vi "Live Modification Dialog.vi"(11 "Front Panel Objects":refnum<vi>[](array[refnum])) -> ()   [LabVIEW 2019, in "LSS.lvlib"]
doc: "This dialog box can be used to help generate style sheets and observe their effect on the user interface. The editor will populate with the default values for each LSS style when an item from \"Available Properties\" is double clicked. \n\n<b>Inputs:</b>\n<b>Front Panel Objects</b> - Although the editor is setup to allow a user to select an active VI to edit, this input can be used to pass in Front Panel Objects if the references are already open when usinng this VI as a pop up dialog."
uses:
  LSS.lvlib
  Controls/Mode.ctl
panel:
  out "Error Out":errorcluster
  in  "Error In":errorcluster
  in  "Color Map":string
  in  "Editable VIs":i32[](listbox)
  in  "HEX":string
  in  "B":u32 max=255
  in  "G":u32 max=255
  in  "R":u32 max=255
  in  "Color Picker":u32(colorbox)
  in  "Clear":bool
  out "Applicable Controls":i32(listbox)
  in  "Available Properties":i32(listbox) caption="Available Properties\n(double click to add)"
  out "More Specific Identifiers":i32(listbox)
  out "More Generic Identifiers":i32(listbox)
  in  "Unique Identifiers":i32(listbox)
  in  "Load":bool
  in  "Save":bool
  in  "Apply":bool
  in  "LSS Editor":string
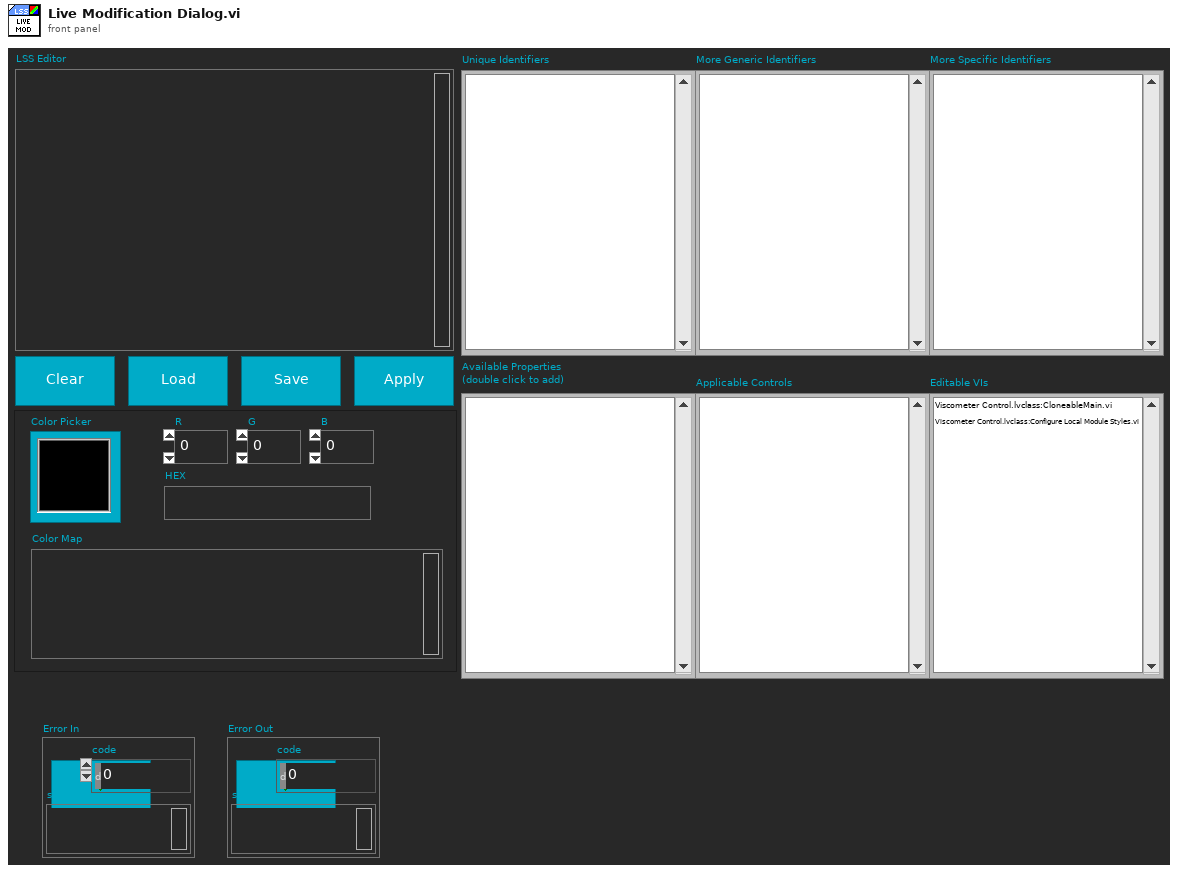
[diagram p1: front panel]
types:
  T1 = typedef "LSS.lvlib/Mode.ctl" = enum16{"Write", "Add", "Read"}
  T2 = typedef "LVPoint32TypeDef.ctl" = cluster{"Horizontal":i32, "Vertical":i32}
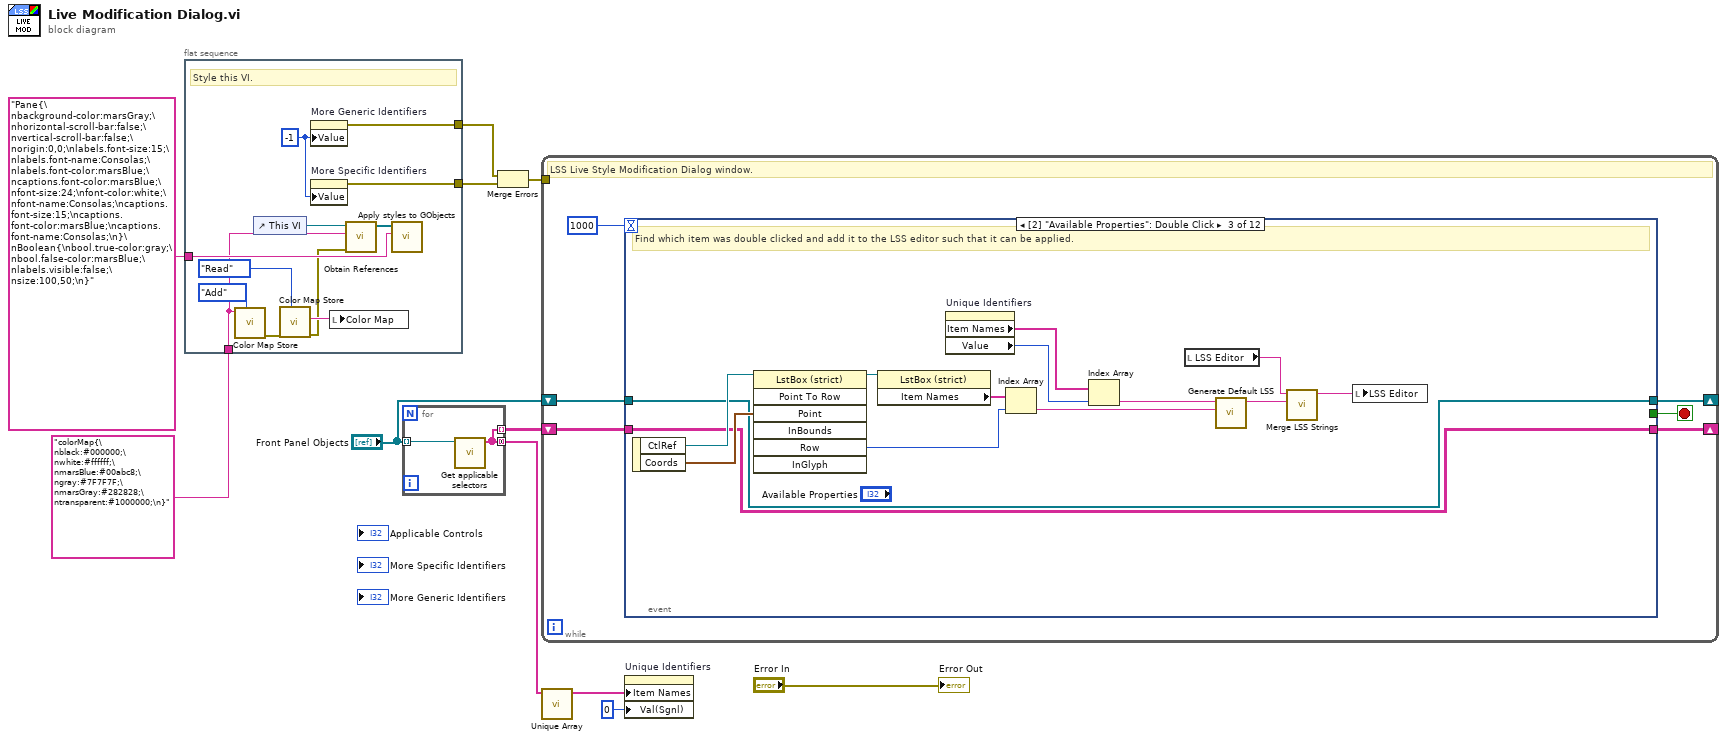
[diagram p0: block diagram]
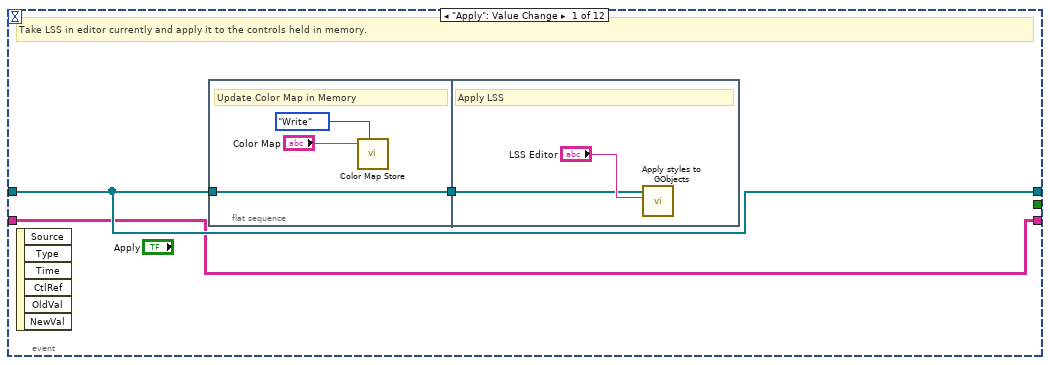
[diagram p2: hidden frame]
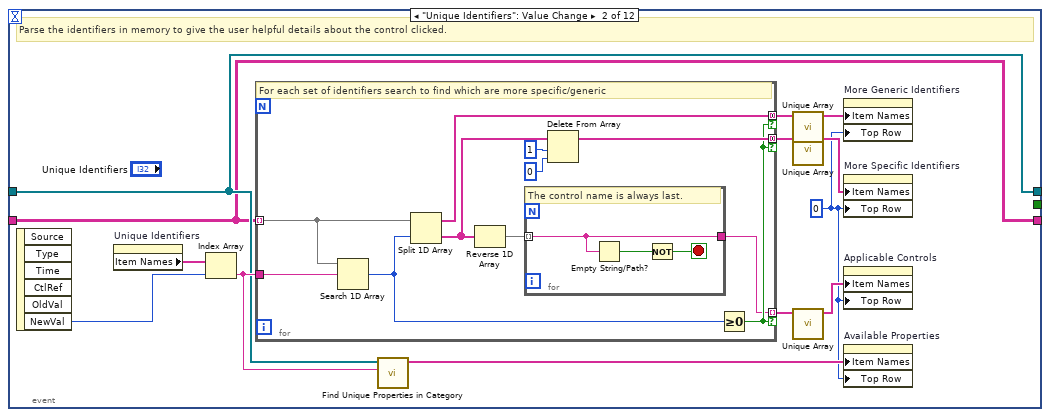
[diagram p3: hidden frame]
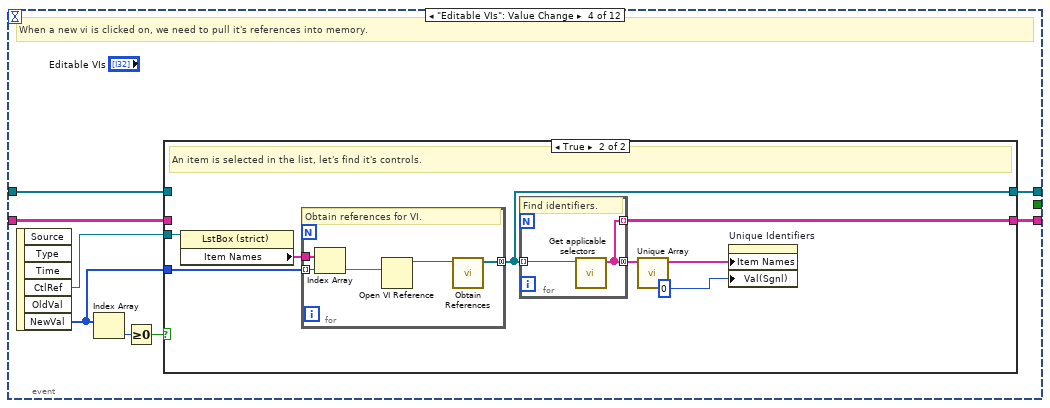
[diagram p4: hidden frame]
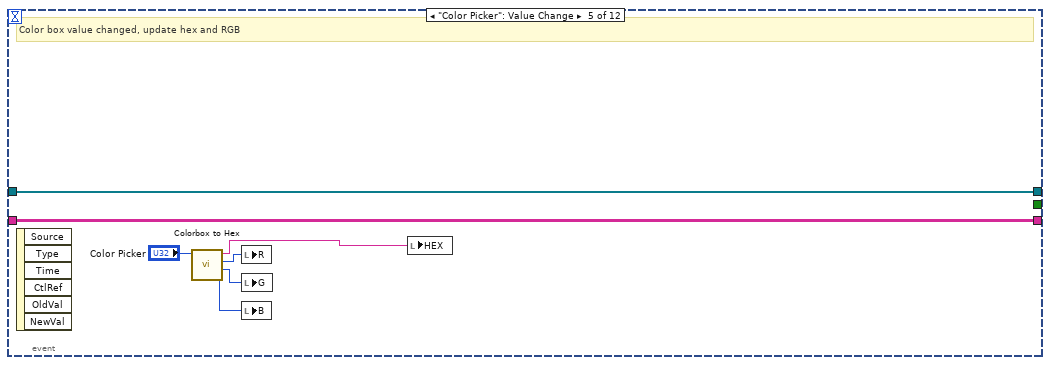
[diagram p6: hidden frame]
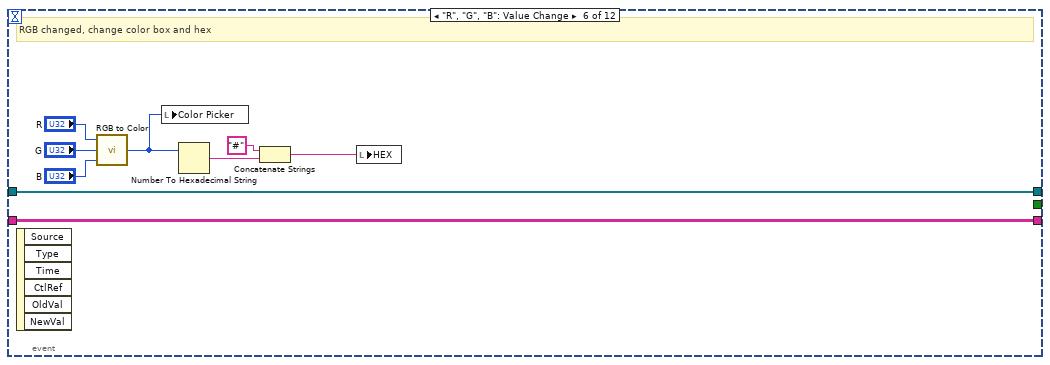
[diagram p7: hidden frame]
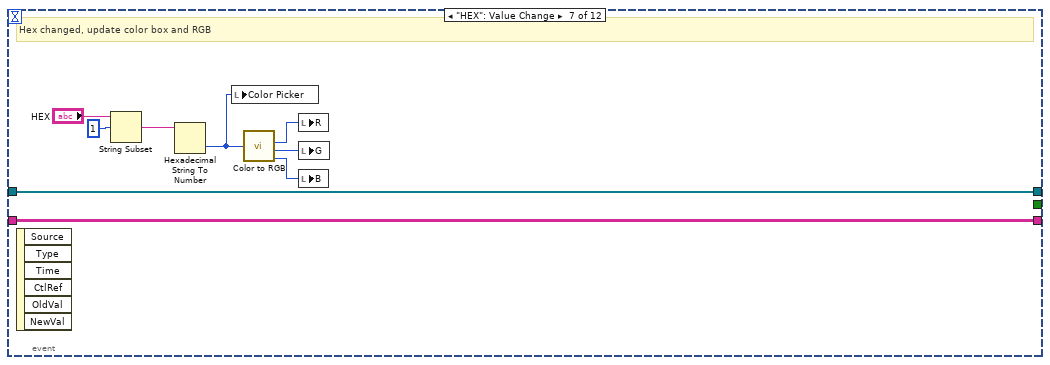
[diagram p8: hidden frame]
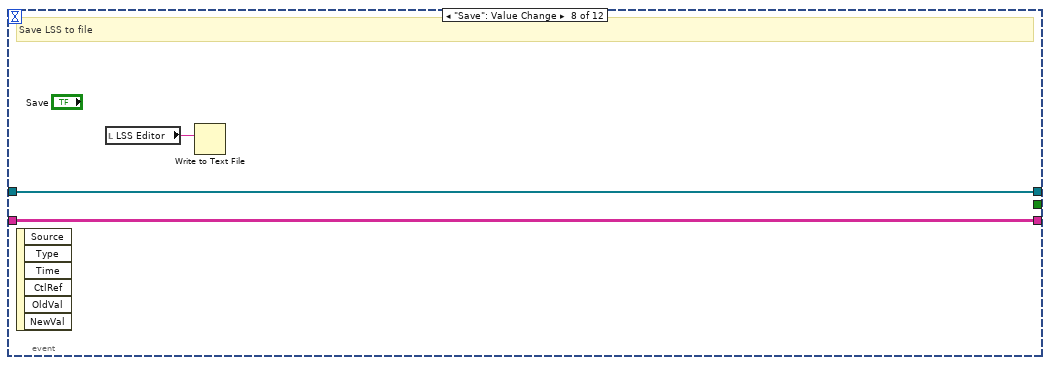
[diagram p9: hidden frame]
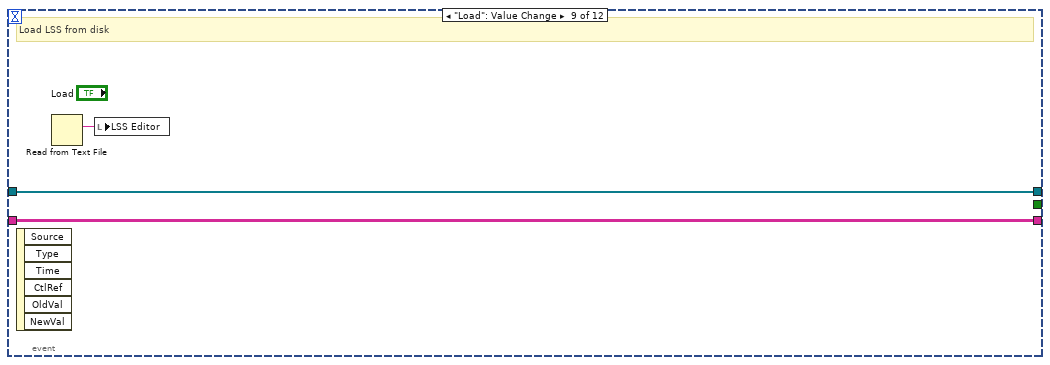
[diagram p10: hidden frame]
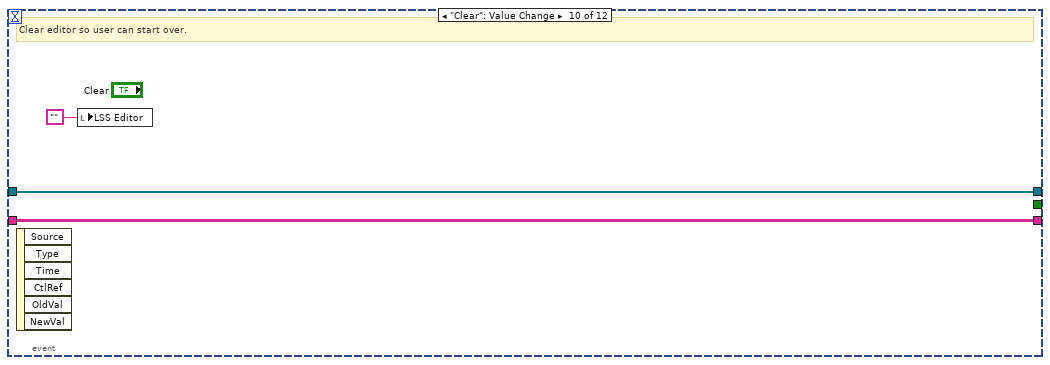
[diagram p11: hidden frame]
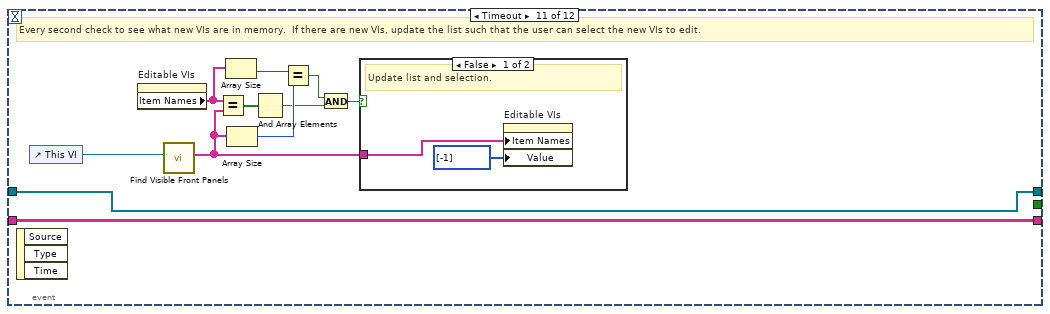
[diagram p12: hidden frame]
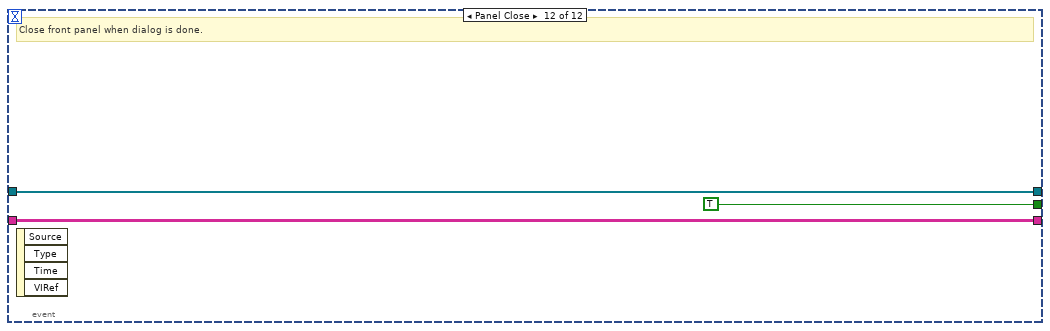
[diagram p14: hidden frame]
diagram:
  n1 = flat-sequence {
    tunnel: [w22] -> w7
    tunnel: [w21] -> w6
    tunnel: "Pane{\nbackground-color:marsGray;\nhorizontal-scroll-bar:false;\nvertical-scroll-bar:false;\norigin:0,0;\nlabels.font-size:15;\nlabels.font-name:Consolas;\nlabels.font-color:marsBlue;\ncaptions.font-color:marsBlue;\nfont-size:24;\nfont-color:white;\nfont-name:Consolas;\ncaptions.font-size:15;\ncaptions.font-color:marsBlue;\ncaptions.font-name:Consolas;\n}\nBoolean{\nbool.true-color:gray;\nbool.false-color:marsBlue;\nlabels.visible:false;\nsize:100,50;\n}" ("String") -> [w18]
    tunnel: "colorMap{\nblack:#000000;\nwhite:#ffffff;\nmarsBlue:#00abc8;\ngray:#7F7F7F;\nmarsGray:#282828;\ntransparent:#1000000;\n}" ("colorMap") -> [w12]
    frame #0 {
      w23 = -1 ("Active Row:Active Row Number")
      # "Style this VI."
      n2 = call "Color Map Store.vi"("Mode"=Mode."Add", "colorMap"=w12) -> ("Error Out"=w14:errorcluster)  [unwired: 7 in, 2 out]
      n3 = control-ref of="This VI"() -> (w20:refnum<vi>)
      n4 = call "Color Map Store.vi"("Mode"=Mode."Read", "Error In"=w14) -> ("Error Out"=w15:errorcluster, "colorMap String"=w16:string)  [unwired: 7 in, 1 out]
      n5 = property on="More Generic Identifiers" class="LstBox (strict)"("Value"=w23) -> (error out=w22:errorcluster)  [unwired: 2 in, 1 out]
      n6 = property on="More Specific Identifiers" class="LstBox (strict)"("Value"=w23) -> (error out=w21:errorcluster)  [unwired: 2 in, 1 out]
      n7 = local write "Color Map"(w16) -> ()
      n8 = call "Obtain References.vi"("Error In"=w15, "colorMap"=w12, "VI in"=w20) -> ("Front Panel Objects"=w19:refnum<vi>[])  [unwired: 7 in, 1 out]
      n9 = call "Apply styles to GObjects.vi"("Style Sheet"=w18, "Front Panel Objects"=w19) -> ()  [unwired: 8 in, 2 out]
    }
  }
  n10 = for {
    tunnel: "Front Panel Objects" -> [w25] mode=indexing
    tunnel: [w24] -> w10 mode=indexing
    tunnel: [w24] -> w9 mode=concatenating
    n11 = call "Get applicable selectors.vi"("GObject"=w25) -> ("Selectors"=w24:string[])  [unwired: 9 in, 1 out]
  }
  n12 = Merge Errors(w7, w6) -> (w5:errorcluster)
  n13 = while {
    tunnel: w5 -> [_]
    shift-right: [w27] -> _
    shift-left: "Front Panel Objects" -> [w31]
    shift-right: [w26] -> _
    shift-left: w10 -> [w29]
    stop <- w30 stop-if-true
    # "LSS Live Style Modification Dialog window."
    n14 = event shown="[2] \"Available Properties\": Double Click" {
      selector: _ -> [_ _ _ _ _ _ _ _ _ _ _ _]
      dyn-events: _ -> [_ _ _ _ _ _ _ _ _ _ _ _]
      timeout: 1000 -> [_ _ _ _ _ _ _ _ _ _ _ _]
      tunnel: w31 -> [w34 w41 w71 w83 w110 w114 w123 w132 w135 w138 w150 w154]
      tunnel: [_ _ _ _ _ _ _ _ _ _ _ TRUE] -> w30
      tunnel: w29 -> [w33 w40 w70 w82 w109 w113 w122 w131 w134 w137 w147 w153]
      tunnel: [w34 w41 w71 w87 w110 w114 w123 w132 w135 w138 w150 w154] -> w27
      tunnel: [w33 w40 w70 w81 w109 w113 w122 w131 w134 w137 w147 w153] -> w26
      event "Apply": Value Change {
        # "Take LSS in editor currently and apply it to the controls held in memory."
        n15 = event-data() -> ()  [unwired: 1 in, 6 out]
        n16 = flat-sequence {
          tunnel: w34 -> [w37]
          tunnel: [w37] -> w32
          tunnel: w32 -> [w38]
          frame #0 {
            # "Update Color Map in Memory"
            n17 = call "Color Map Store.vi"("Mode"=Mode."Write", "colorMap"="Color Map") -> ()  [unwired: 7 in, 3 out]
          }
          frame #1 {
            # "Apply LSS"
            n18 = call "Apply styles to GObjects.vi"("Style Sheet"="LSS Editor", "Front Panel Objects"=w38) -> ()  [unwired: 8 in, 2 out]
          }
        }
      }
      event "Unique Identifiers": Value Change {
        w42 = 0 ("Top Row")
        # "Parse the identifiers in memory to give the user helpful details about the control clicked."
        n19 = event-data() -> ("NewVal"=w51:i32)  [unwired: 1 in, 5 out]
        n20 = property on="Unique Identifiers" class="LstBox (strict)"() -> ("Item Names"=w52:string[])  [unwired: 2 in, 2 out]
        n21 = Index Array(array=w52, index=w51) -> (element=w45:string)
        n22 = for {
          tunnel: w40 -> [w62] mode=indexing
          tunnel: w45 -> [w63]
          tunnel: [w61] -> w49 mode=concatenating if=w56
          tunnel: [w59] -> w47 mode=concatenating if=w56
          tunnel: [w53] -> w46 mode=indexing if=w56
          # "For each set of identifiers search to find which are more specific/generic"
          n23 = Search 1D Array(1D array=w62, element=w63) -> (index of element=w60:i32)  [unwired: 1 in]
          n24 = Split 1D Array(array=w62, index=w60) -> (first subarray=w61:string[], second subarray=w55:string[])
          n25 = Reverse 1D Array(array=w55) -> (reversed array=w54:string[])
          n26 = for {
            tunnel: w54 -> [w66] mode=indexing
            tunnel: [w66] -> w53
            stop <- w64 stop-if-true
            # "The control name is always last."
            n27 = Empty String/Path?(string/path=w66) -> (empty?=w65:bool)
            n28 = Not(x=w65) -> (.not. x?=w64:bool)
          }
          n29 = Delete From Array(array=w55, length=1, index=0) -> (array with subset deleted=w59:string[])  [unwired: 1 out]
          n30 = Greater Or Equal To 0?(x=w60) -> (x >= 0?=w56:bool)
        }
        n31 = call "Find Unique Properties in Category.vi"("Unique Identifier"=w45, "Front Panel Objects"=w41) -> ("Unique Properties in Category"=w44:string[])  [unwired: 9 in]
        n32 = call "Unique Array.vi"("Array"=w49) -> ("Unique Array"=w48:string[])  [unwired: 10 in]
        n33 = call "Unique Array.vi"("Array"=w47) -> ("Unique Array"=w50:string[])  [unwired: 10 in]
        n34 = call "Unique Array.vi"("Array"=w46) -> ("Unique Array"=w43:string[])  [unwired: 10 in]
        n35 = property on="More Generic Identifiers" class="LstBox (strict)"("Item Names"=w48, "Top Row"=w42) -> ()  [unwired: 2 in, 2 out]
        n36 = property on="More Specific Identifiers" class="LstBox (strict)"("Item Names"=w50, "Top Row"=w42) -> ()  [unwired: 2 in, 2 out]
        n37 = property on="Applicable Controls" class="LstBox (strict)"("Item Names"=w43, "Top Row"=w42) -> ()  [unwired: 2 in, 2 out]
        n38 = property on="Available Properties" class="LstBox (strict)"("Item Names"=w44, "Top Row"=w42) -> ()  [unwired: 2 in, 2 out]
      }
      event "Available Properties": Double Click {
        # "Find which item was double clicked and add it to the LSS editor such that it can be applied."
        n39 = event-data() -> ("CtlRef"=w80:refnum<vi>, "Coords"=w79:T2)  [unwired: 1 in]
        n40 = invoke class="LstBox (strict)" method="Point To Row"(reference=w80, "Point"=w79) -> (reference out=w78:refnum<vi>, "Row"=w76:i32)  [unwired: 5 in, 5 out]
        n41 = property class="LstBox (strict)"(reference=w78) -> ("Item Names"=w77:string[])  [unwired: 1 in, 2 out]
        n42 = property on="Unique Identifiers" class="LstBox (strict)"() -> ("Item Names"=w75:string[], "Value"=w74:i32)  [unwired: 2 in, 2 out]
        n43 = Index Array(array=w77, index=w76) -> (element=w72:string)
        n44 = Index Array(array=w75, index=w74) -> (element=w73:string)
        n45 = local read "LSS Editor"() -> (w69:string)
        n46 = call "Generate Default LSS.vi"("Property"=w72, "Identifier"=w73) -> ("LSS Format"=w68:string)  [unwired: 9 in]
        n47 = call "Merge LSS Strings.vi"("Merge String"=w68, "LSS Before"=w69) -> ("LSS After"=w67:string)  [unwired: 9 in]
        n48 = local write "LSS Editor"(w67) -> ()
      }
      event "Editable VIs": Value Change {
        # "When a new vi is clicked on, we need to pull it's references into memory."
        n49 = event-data() -> ("CtlRef"=w88:refnum<vi>, "NewVal"=w85:i32[])  [unwired: 1 in, 4 out]
        n50 = Index Array(array=w85) -> (element=w86:i32)  [unwired: 1 in]
        n51 = Greater Or Equal To 0?(x=w86) -> (x >= 0?=w84:bool)
        n52 = case shown="True" w84 {
          tunnel: w88 -> [_ w98]
          tunnel: [w90 w95] -> w87
          tunnel: w85 -> [_ w96]
          tunnel: w83 -> [w90 _]
          tunnel: w82 -> [w89 _]
          tunnel: [w89 w94] -> w81
          frame False {
            # "Nothing selected in list, it was just reset, do nothing."
          }
          frame True {
            # "An item is selected in the list, let's find it's controls."
            n53 = property class="LstBox (strict)"(reference=w98) -> ("Item Names"=w97:string[])  [unwired: 1 in, 2 out]
            n54 = for {
              tunnel: w96 -> [w104] mode=indexing
              tunnel: w97 -> [w105]
              tunnel: [w101] -> w95 mode=concatenating
              # "Obtain references for VI."
              n55 = Index Array(array=w105, index=w104) -> (element=w103:string)
              n56 = Open VI Reference(vi path=w103) -> (vi reference=w102:refnum<vi>)  [unwired: 5 in, 1 out]
              n57 = call "Obtain References.vi"("VI in"=w102) -> ("Front Panel Objects"=w101:refnum<vi>[])  [unwired: 9 in, 1 out]
            }
            n58 = for {
              tunnel: w95 -> [w100] mode=indexing
              tunnel: [w99] -> w94 mode=indexing
              tunnel: [w99] -> w92 mode=concatenating
              # "Find identifiers."
              n59 = call "Get applicable selectors.vi"("GObject"=w100) -> ("Selectors"=w99:string[])  [unwired: 9 in, 1 out]
            }
            n60 = call "Unique Array.vi"("Array"=w92) -> ("Unique Array"=w91:string[])  [unwired: 10 in]
            n61 = property on="Unique Identifiers" class="LstBox (strict)"("Item Names"=w91, "Val(Sgnl)"=0 ("Value (Signaling)")) -> ()  [unwired: 2 in, 2 out]
          }
        }
      }
      event "Color Picker": Value Change {
        # "Color box value changed, update hex and RGB"
        n62 = event-data() -> ()  [unwired: 1 in, 6 out]
        n63 = call "Colorbox to Hex.vi"("Color Picker"="Color Picker") -> ("B"=w106:u8, "G"=w107:u8, "R"=w108:u8, "HEx String"=w111:string)  [unwired: 7 in]
        n64 = local write "R"(w108) -> ()
        n65 = local write "G"(w107) -> ()
        n66 = local write "B"(w106) -> ()
        n67 = local write "HEX"(w111) -> ()
      }
      event "R", "G", "B": Value Change {
        # "RGB changed, change color box and hex"
        n68 = event-data() -> ()  [unwired: 1 in, 6 out]
        n69 = call <vilib>:"RGB to Color.vi"("B"="B", "G"="G", "R"="R") -> ("Color"=w116:u32)
        n70 = local write "Color Picker"(w116) -> ()
        n71 = Number To Hexadecimal String(2:w116) -> (0:w118:string)  [unwired: 1 in]
        n72 = Concatenate Strings("#" ("string"), w118) -> (w115:string)
        n73 = local write "HEX"(w115) -> ()
      }
      event "HEX": Value Change {
        # "Hex changed, update color box and RGB"
        n74 = event-data() -> ()  [unwired: 1 in, 6 out]
        n75 = String Subset(string="HEX", offset (0)=1) -> (substring=w128:string)  [unwired: 1 in]
        n76 = Hexadecimal String To Number(string=w128) -> (number=w124:u32)  [unwired: 2 in, 1 out]
        n77 = local write "Color Picker"(w124) -> ()
        n78 = call <vilib>:"Color to RGB.vi"("Color"=w124) -> ("R"=w127:u8, "G"=w126:u8, "B"=w125:u8)  [unwired: 1 out]
        n79 = local write "R"(w127) -> ()
        n80 = local write "G"(w126) -> ()
        n81 = local write "B"(w125) -> ()
      }
      event "Save": Value Change {
        # "Save LSS to file"
        n82 = event-data() -> ()  [unwired: 1 in, 6 out]
        n83 = local read "LSS Editor"() -> (w133:string)
        n84 = Write to Text File(text=w133) -> ()  [unwired: 3 in, 3 out]
      }
      event "Load": Value Change {
        # "Load LSS from disk"
        n85 = event-data() -> ()  [unwired: 1 in, 6 out]
        n86 = Read from Text File() -> (text=w136:string)  [unwired: 4 in, 3 out]
        n87 = local write "LSS Editor"(w136) -> ()
      }
      event "Clear": Value Change {
        # "Clear editor so user can start over."
        n88 = event-data() -> ()  [unwired: 1 in, 6 out]
        n89 = local write "LSS Editor"("" ("New CSS to Apply")) -> ()
      }
      event Timeout {
        # "Every second check to see what new VIs are in memory.  If there are new VIs, update the list such that the user can select the new VIs to edit."
        n90 = event-data() -> ()  [unwired: 1 in, 3 out]
        n91 = control-ref of="This VI"() -> (w148:refnum<vi>)
        n92 = property on="Editable VIs" class="LstBox (strict)"() -> ("Item Names"=w146:string[])  [unwired: 2 in, 2 out]
        n93 = call "Find Visible Front Panels.vi"("This VI"=w148) -> ("Running VIs"=w145:string[])  [unwired: 9 in, 1 out]
        n94 = Equal?(x=w146, y=w145) -> (x = y?=w149:bool[])
        n95 = Array Size(array=w146) -> (size(s)=w144:i32)
        n96 = Array Size(array=w145) -> (size(s)=w143:i32)
        n97 = And Array Elements(Boolean array=w149) -> (logical AND=w142:bool)
        n98 = Equal?(x=w144, y=w143) -> (x = y?=w141:bool)
        n99 = And(x=w141, y=w142) -> (x .and. y?=w140:bool)
        n100 = case shown="False" w140 {
          tunnel: w145 -> [w152 _]
          frame False {
            # "Update list and selection."
            n101 = property on="Editable VIs" class="LstBox (strict)"("Item Names"=w152, "Value"=i32[] [-1] ("Editable VIs")) -> ()  [unwired: 2 in, 2 out]
          }
          frame True {
            # "No change, do nothing."
          }
        }
      }
      event Panel Close {
        # "Close front panel when dialog is done."
        n102 = event-data() -> ()  [unwired: 1 in, 4 out]
      }
    }
  }
  n103 = call "Unique Array.vi"("Array"=w9) -> ("Unique Array"=w8:string[])  [unwired: 10 in]
  n104 = property on="Unique Identifiers" class="LstBox (strict)"("Item Names"=w8, "Val(Sgnl)"=0 ("Value (Signaling)")) -> ()  [unwired: 2 in, 2 out]
  "Error Out" <- "Error In"
